vi "rot_proc.vi"(0 "Euler Angles":dbl[][](array[numeric]) format="%.2f", 7 "Error in":errorcluster) -> (13 "Error out":errorcluster, 14 "Rotation Vectors":dbl[][](array[numeric])=[[-0.73760986328125, -3.32122802734375, 5.82550048828125, -1.02630615234375, -0.74188232421875], [-3.3197021484375, 5.81512451171875, 1.1328125, 0.05096435546875, -0.73577880859375], [-3.3209228515625, 5.8258056640625, -1.03668212890625, -0.740966796875, -3.31939697265625], [5.81573486328125, 1.14288330078125, 0.0537109375, -0.7366943359375, -3.32061767578125], [5.8294677734375, -1.03912353515625, -0.7415771484375, -3.32000732421875, 5.8197021484375]] format="%.2f")   [LabVIEW 2016]
panel:
  # "DATA PROCESSOR"
  # "This program reads a calibration and data file\nto produce Rotation Vectors and Velocity vectors \nin space co-ordinates.\nBy Americo Aniello Migliaccio   v1.0     21 Jul 1999"
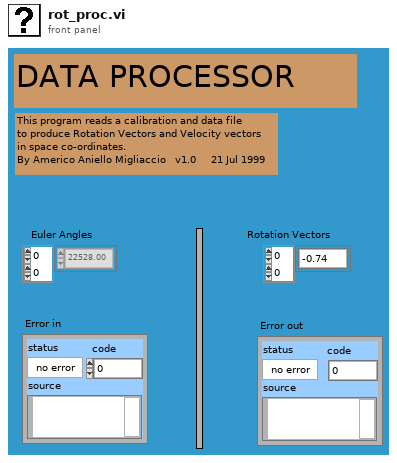
[diagram p1: front panel]
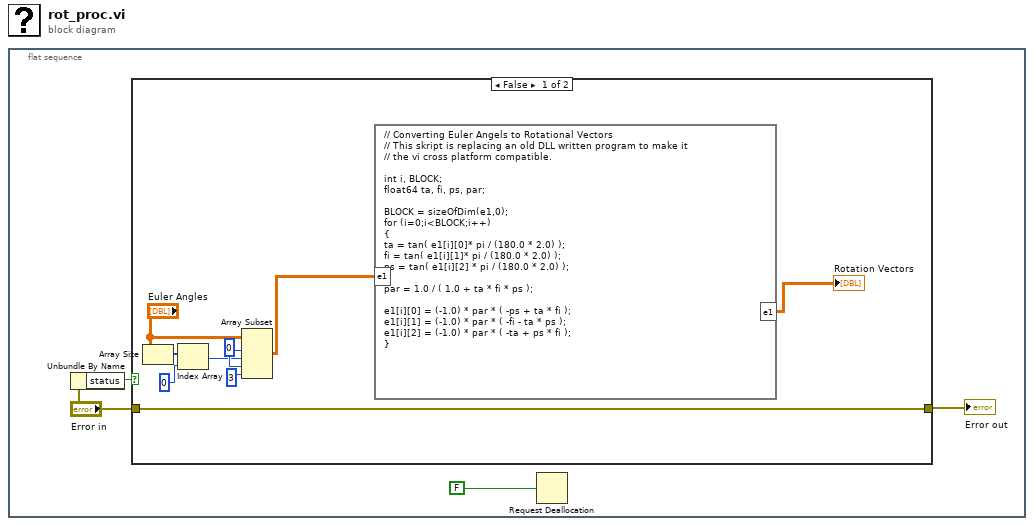
[diagram p0: block diagram]
diagram:
  n1 = flat-sequence {
    frame #0 {
      n2 = Unbundle By Name("Error in") -> ("status"=w4:bool)
      n3 = case shown="False" w4 {
        tunnel: "Error in" -> [w7 w14]
        tunnel: [w7 w14] -> w2
        frame False {
          w11 = 0
          n4 = Array Size(array="Euler Angles") -> (size(s)=w8:i32[])
          n5 = Index Array(array=w8, index=0) -> (element=w10:i32)
          n6 = Array Subset(array="Euler Angles", index (row)=w11, length (row)=w10, index (col)=w11, length (col)=3) -> (w6:dbl[][])
          n7 = formula code="// Converting Euler Angels to Rotational Vectors\n// This skript is replacing an old DLL written program to make it\n// the vi cross platform compatible.\n\nint i, BLOCK;\nfloat64 ta, fi, ps, par;\n\nBLOCK = sizeOfDim(e1,0);\nfor (i=0;i<BLOCK;i++)\n{\nta = tan( e1[i][0]* pi / (180.0 * 2.0) ); \nfi = tan( e1[i][1]* pi / (180.0 * 2.0) );    \nps = tan( e1[i][2] * pi / (180.0 * 2.0) );\n\npar = 1.0 / ( 1.0 + ta * fi * ps );\n\ne1[i][0] = (-1.0) * par * ( -ps + ta * fi );\ne1[i][1] = (-1.0) * par * ( -fi - ta * ps );\ne1[i][2] = (-1.0) * par * ( -ta + ps * fi );\n}"("e1"=w6) -> ("e1"=→"Rotation Vectors":dbl[][])
        }
        frame True {
        }
      }
      "Error out" <- w2
      n8 = Request Deallocation(FALSE ("flag")) -> ()
    }
  }
